vi "Resume Processing.vi"(8 "error in (no error)":errorcluster, 10 "Queue in":refnum<queue>) -> (0 "error out":errorcluster)   [LabVIEW 2023, in "HAF.lvlib" / "TestProcessor.lvclass"]
doc: "Resumes processing Command Directors after a Pause."
uses:
  TestProcessor.lvclass
  TestProcessor.lvclass/TestProcessor.ctl
  HAF.lvlib
  All Internal Message Ids.ctl
  Message.ctl
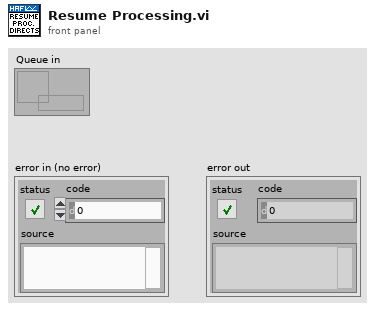
[diagram p1: front panel]
types:
  T1 = typedef "HAF.lvlib/All Internal Message Ids.ctl" = cluster{"Initialise":string, "Process":string, "Continue":string, "Done":string, "Pause":string, "Resume":string, "Stop":string, "Exit":string}
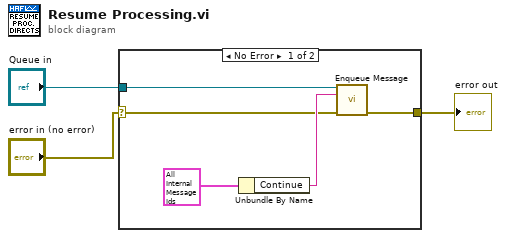
[diagram p0: block diagram]
diagram:
  n1 = case shown="No Error" "error in (no error)" {
    selector: "error in (no error)" -> [w4 w9]
    tunnel: [w8 w9] -> w3
    tunnel: "Queue in" -> [w5 _]
    frame No Error {
      n2 = Unbundle By Name(T1 {"Initialise"="Initialise", "Process"="Process", "Continue"="Continue", "Done"="Done", "Pause"="Pause", "Resume"="Resume", "Stop"="Stop", "Exit"="Exit"} ("Message Ids")) -> ("Continue"=w7:string)
      n3 = call "Enqueue Message.vi"("Message Queue In"=w5, "Message Id"=w7, "error in (no error)"=w4) -> ("error out"=w8:errorcluster)  [unwired: 11 in, 1 out]
    }
    frame Error {
    }
  }
  "error out" <- w3
